vi "write_samples_per_sec.vi"(0 "Byte Stream File in":T1, 1 "task in":refnum<k21>, 2 "Volume":dbl(slide) scale=0.0..0.5, 3 "Playback speed":dbl(knob) scale=0.25..2.0, 5 "Sample offset":u64, 9 "Samples per channel":dbl, 11 "error in":errorcluster) -> (4 "Refnum out":refnum<k21>, 6 "next_offset":u64, 8 "data out":waveform(dbl), 10 "end of file?":bool, 14 "duration":u32, 15 "error out":errorcluster)   [LabVIEW 2022 SP3]
uses:
  <vilib>/sound2/lvsound2.llb/Sound File Refnum.ctl
  <vilib>/sound2/lvsound2.llb/Sound File Position.ctl
  <vilib>/DAQmx/write.llb/DAQmx Write (Analog Wfm 1Chan NSamp).vi
  <vilib>/sound2/lvsound2.llb/Sound File Read (DBL).vi
  <vilib>/DAQmx/miscellaneous.llb/DAQmx Fill In Error Info.vi
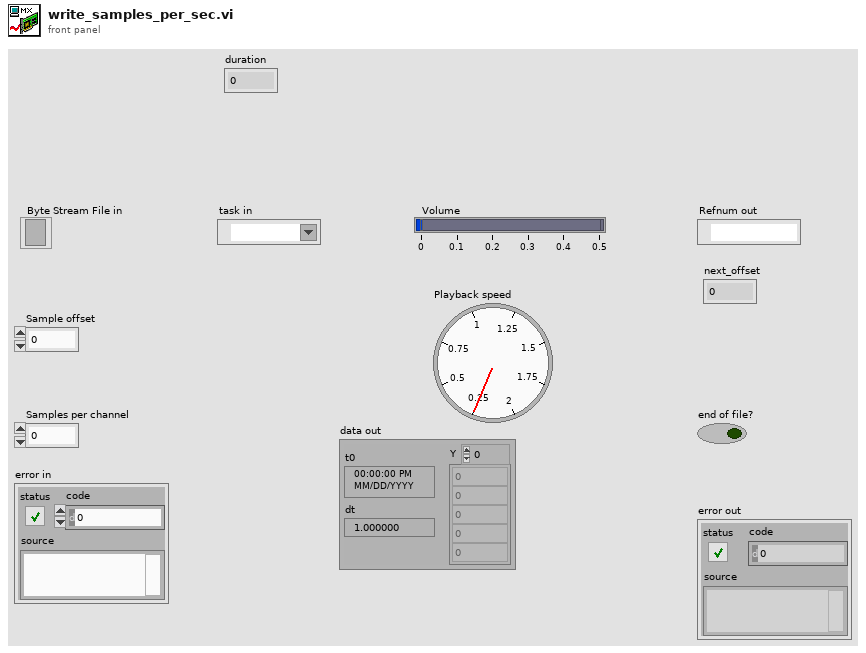
[diagram p1: front panel]
types:
  T1 = typedef "Sound File Refnum.ctl" = refnum<file>
  T2 = typedef "Sound File Position.ctl" = u16
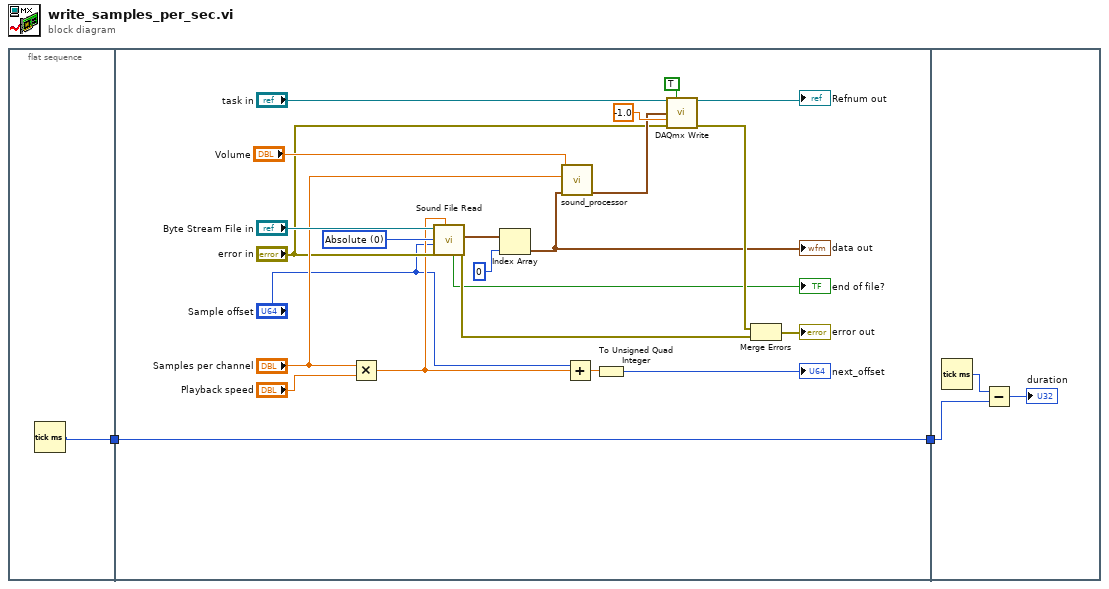
[diagram p0: block diagram]
diagram:
  n1 = flat-sequence {
    tunnel: [w3] -> w1
    tunnel: [w4] -> w2
    tunnel: w1 -> [w4]
    tunnel: w2 -> [w28]
    frame #0 {
      n2 = Tick Count (ms)() -> (millisecond timer value=w3:u32)
    }
    frame #1 {
      w15 = T2 0 items=["Absolute"=0, "Relative"=2] ("position mode")
      n3 = Multiply(x="Samples per channel", y="Playback speed") -> (x*y=w8:dbl)
      n4 = call-poly <vilib>:"Sound File Read.vi"("number of samples/ch (-1: all)"=w8, "error in (no error)"="error in", "position offset"="Sample offset", "position mode"=w15, "sound file refnum"="Byte Stream File in") -> ("error out"=w18:errorcluster, "data"=w20:waveform(dbl)[], "end of file?"=→"end of file?":bool)  [unwired: 2 in, 2 out]
      n5 = Index Array(array=w20, index=0) -> (element=w9:waveform(dbl))
      "data out" <- w9
      n6 = call "sound_processor.vi"("data in"=w9, "Target samples per channel"="Samples per channel", "Volume"="Volume") -> ("data out"=w12:waveform(dbl))  [unwired: 8 in]
      n7 = Add(x="Sample offset", y=w8) -> (x+y=w6:dbl)
      n8 = To Unsigned Quad Integer(1:w6) -> (0:→"next_offset":u64)
      n9 = call-poly <vilib>:"DAQmx Write.vi"("task/channels in"="task in", "auto start"=TRUE, "data"=w12, "timeout"=-1.0, "error in"="error in") -> ("task out"=→"Refnum out":refnum<k21>, "error out"=w22:errorcluster)  [unwired: 8 in, 1 out]
      n10 = Merge Errors(w22, w18) -> (→"error out":errorcluster)
    }
    frame #2 {
      n11 = Tick Count (ms)() -> (millisecond timer value=w29:u32)
      n12 = Subtract(x=w29, y=w28) -> (x-y=→"duration":u32)
    }
  }
